vi "Update Out of Date.vi"(8 "error in (no error)":errorcluster, 11 "Message Maker in":refnum<class "Message Maker.lvclass">) -> (0 "error out":errorcluster, 3 "Message Maker out":refnum<class "Message Maker.lvclass">)   [LabVIEW 2023, in "Message Maker.lvclass"]
uses:
  Message Maker.lvclass
  Message Maker.lvclass/Message Maker.ctl
  Message Status.ctl
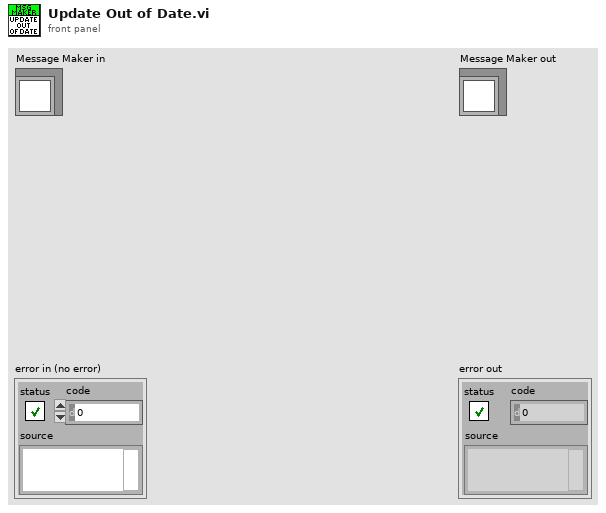
[diagram p1: front panel]
types:
  T1 = typedef "Message Maker.lvclass/Message Status.ctl" = enum16{"Message Not Created", "Message Out of Date", "Message OK", "Never update"}
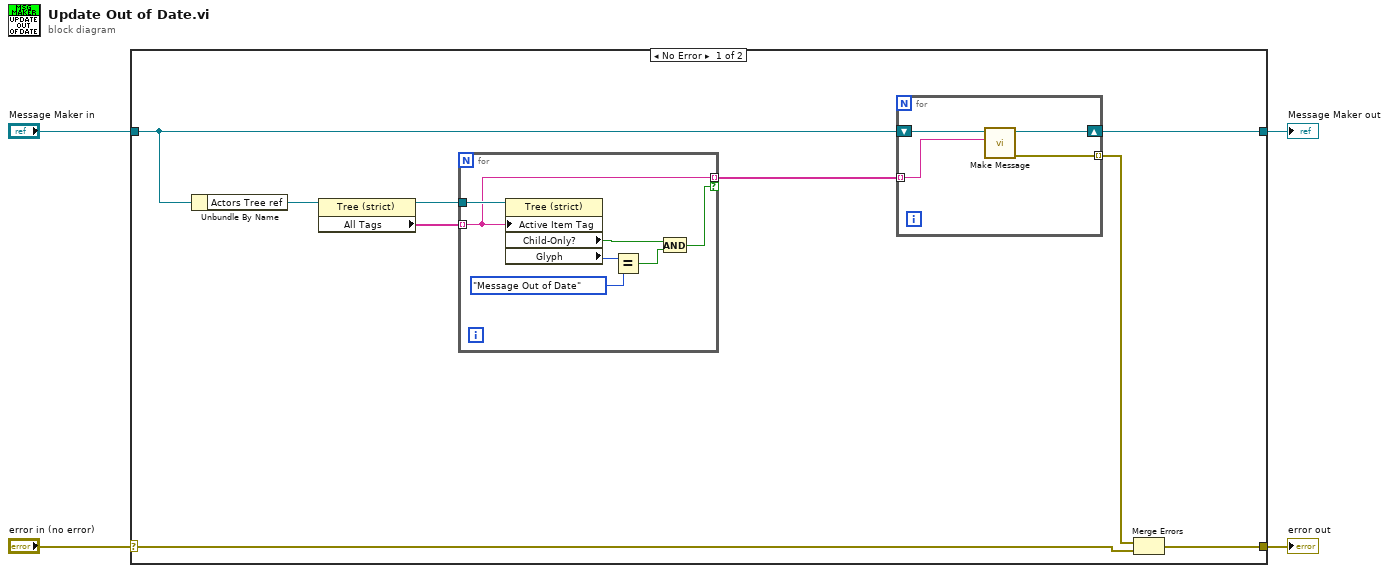
[diagram p0: block diagram]
diagram:
  n1 = case shown="No Error" "error in (no error)" {
    selector: "error in (no error)" -> [w5 w26]
    tunnel: [w6 w26] -> w3
    tunnel: [w13 w25] -> w1
    tunnel: "Message Maker in" -> [w12 w25]
    frame No Error {
      n2 = Unbundle By Name(w12) -> ("Actors Tree ref"=w11:refnum<vi>)
      n3 = property class="Tree (strict)"(reference=w11) -> (reference out=w9:refnum<vi>, "All Tags"=w10:string[])  [unwired: 1 in, 1 out]
      n4 = for {
        tunnel: w10 -> [w15] mode=indexing
        tunnel: w9 -> [w20]
        tunnel: [w15] -> w8 mode=indexing if=w14
        n5 = property class="Tree (strict)"(reference=w20, "Active Item Tag"=w15) -> ("Child-Only?"=w16:bool, "Glyph"=w19:i32)  [unwired: 1 in, 2 out]
        n6 = Equal?(x=w19, y=Message_Status."Message Out of Date" ("Enum")) -> (x = y?=w17:bool)
        n7 = And(x=w16, y=w17) -> (x .and. y?=w14:bool)
      }
      n8 = for {
        shift-right: [w23] -> w13
        shift-left: w12 -> [w24]
        tunnel: w8 -> [w22] mode=indexing
        tunnel: [w21] -> w7 mode=indexing
        n9 = call "Make Message.vi"("Method Qualified Name"=w22, "Message Maker in"=w24) -> ("error out"=w21:errorcluster, "Message Maker out"=w23:refnum<class "Message Maker.lvclass">)  [unwired: 8 in]
      }
      n10 = Merge Errors(w7, w5) -> (w6:errorcluster)
    }
    frame Error {
    }
  }
  "error out" <- w3
  "Message Maker out" <- w1
